vi "Calculate AI param.vi"(11 "Status":T1 {"Setting"."X Pos." scale=-5.0..5.0; "Setting"."Y Pos." scale=-5.0..5.0}) -> (2 "# samples per channel":i32, 3 "# channels per frame":i32)   [LabVIEW 2013]
uses:
  init & communication/init-status.ctl
  init & communication/Setting.ctl
  init & communication/event-package.ctl
  init & communication/Event1.ctl
  init & communication/data-package.ctl
  init & communication/Event.ctl
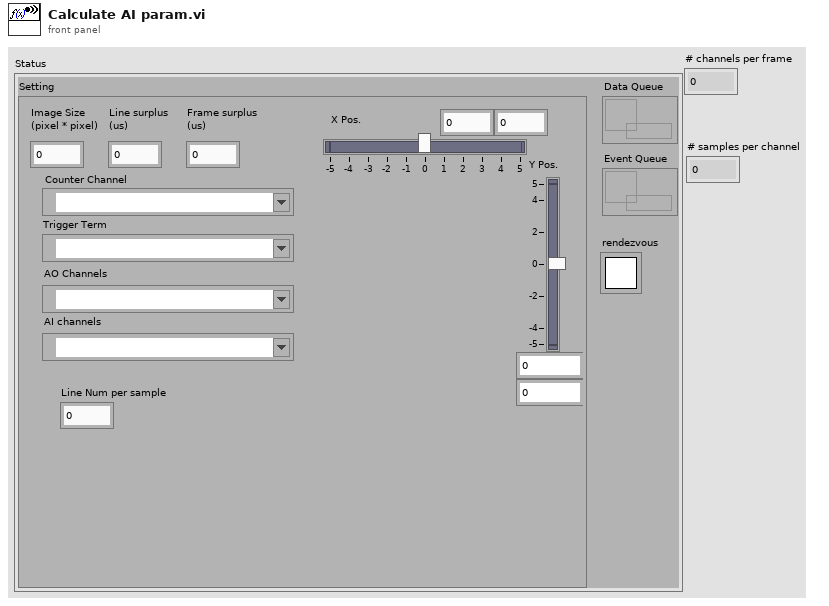
[diagram p1: front panel]
types:
  T1 = typedef "init-status.ctl" = cluster{"Setting":T2, "Event Queue":refnum<queue>, "Data Queue":refnum<queue>, "rendezvous":T3}
  T2 = typedef "Setting.ctl" = cluster{"Image Size\n(pixel * pixel)":i32, "Counter Channel":tag, "Trigger Term":tag, "AO Channels":tag, "Y Pos.":cluster{dbl, dbl}, "X Pos.":cluster{dbl, dbl}, "Line surplus\n(us)":i32, "Frame surplus\n(us)":i32, "AI channels":tag, "Line Num per sample":i32}
  T3 = typedef "Rendezvous RefNum" = refnum<k1>
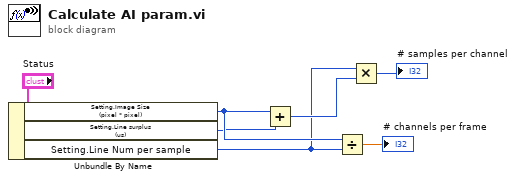
[diagram p0: block diagram]
diagram:
  n1 = Unbundle By Name("Status") -> ("Setting.Image Size\n(pixel * pixel)"=w5:i32, "Setting.Line surplus\n(us)"=w4:i32, "Setting.Line Num per sample"=w2:i32)
  n2 = Add(x=w5, y=w4) -> (x+y=w3:i32)
  n3 = Divide(x=w5, y=w2) -> (x/y=→"# channels per frame":dbl)
  n4 = Multiply(x=w2, y=w3) -> (x*y=→"# samples per channel":i32)
